vi "receiveDCAStats.vi"(8 "error in (no error)":errorcluster, 11 "ILC in":refnum<class "ILC.lvclass">) -> (0 "error out":errorcluster, 1 "Version":string, 2 "Serial Number":string, 3 "ILC out":refnum<class "ILC.lvclass">)   [LabVIEW 2015, in "ILCCommon.lvlib" / "ILC.lvclass"]
uses:
  <userlib>/Common/ILC/ILC/ILC.lvclass
  <userlib>/Common/ILC/ILCModelTypedefs/FinalDelimiter.ctl
  <userlib>/Common/ILC/ILCModelTypedefs/ILCModelTypedefs.lvlib
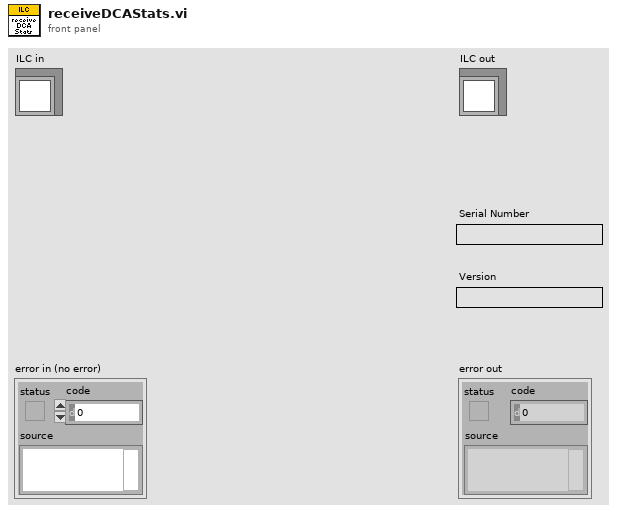
[diagram p1: front panel]
types:
  T1 = typedef "ILCCommon.lvlib/ILCModelTypedefs.lvlib/FinalDelimiter.ctl" = enum16{",", "<CR><LF>"}
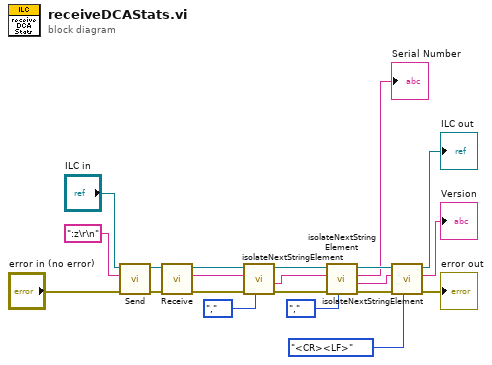
[diagram p0: block diagram]
diagram:
  n1 = call-dynamic "Send.vi"("error in (no error)"="error in (no error)", "Message"=":z\r\n", "ILC in"="ILC in") -> ("error out"=w14:errorcluster, "ILC out"=w15:refnum<class "ILC.lvclass">)  [unwired: 7 in]
  n2 = call-dynamic "Receive.vi"("error in (no error)"=w14, "ILC in"=w15) -> ("error out"=w3:errorcluster, "Response"=w5:string, "ILC out"=w7:refnum<class "ILC.lvclass">)  [unwired: 7 in]
  n3 = call <userlib>:"isolateNextStringElement.vi"("Final Delimiter"=FinalDelimiter.",", "error in (no error)"=w3, "inputString"=w5, "ILC in"=w7) -> ("error out"=w2:errorcluster, "remainingString"=w4:string, "ILC out"=w6:refnum<class "ILC.lvclass">)  [unwired: 4 in, 1 out]
  n4 = call <userlib>:"isolateNextStringElement.vi"("Final Delimiter"=FinalDelimiter.",", "error in (no error)"=w2, "inputString"=w4, "ILC in"=w6) -> ("error out"=w16:errorcluster, "remainingString"=w19:string, "extractedSegment"=→"Serial Number":string, "ILC out"=w18:refnum<class "ILC.lvclass">)  [unwired: 4 in]
  n5 = call <userlib>:"isolateNextStringElement.vi"("Final Delimiter"=FinalDelimiter."<CR><LF>", "error in (no error)"=w16, "inputString"=w19, "ILC in"=w18) -> ("error out"=→"error out":errorcluster, "extractedSegment"=→"Version":string, "ILC out"=→"ILC out":refnum<class "ILC.lvclass">)  [unwired: 4 in, 1 out]
